vi "Motion Plot sub_VI.vi"(8 "Motion Parameters":T2={"Decel Time (s)"=0.0, "Accel Time (s)"=0.0, "Total Time (s)"=0.0, "Max Accel (mm/s^2)"=0.0, "Max Decel (mm/s^2)"=0.0, "Time step (s)"=0.01} {"Time step (s)" min=0.001}) -> (0 "Motion Points":T1, 1 "Accel Array":dbl[](graph), 2 "Velocity Array":dbl[](graph), 3 "Displacement Array":dbl[](graph), 4 "V max (mm/s)":dbl, 5 "Dist max (mm)":dbl)   [LabVIEW 2017]
panel:
  # "Use 0.01s"
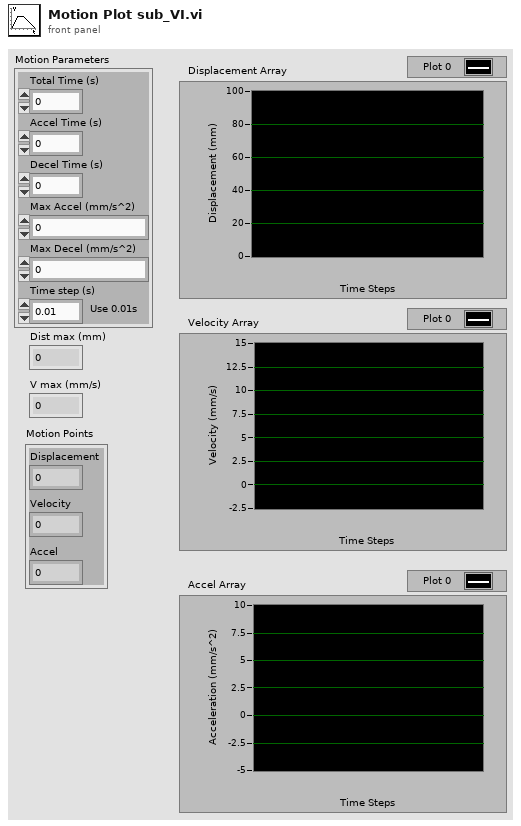
[diagram p1: front panel]
types:
  T1 = cluster{"Accel":dbl, "Velocity":dbl, "Displacement":dbl}
  T2 = cluster{"Decel Time (s)":dbl, "Accel Time (s)":dbl, "Total Time (s)":dbl, "Max Accel (mm/s^2)":dbl, "Max Decel (mm/s^2)":dbl, "Time step (s)":dbl}
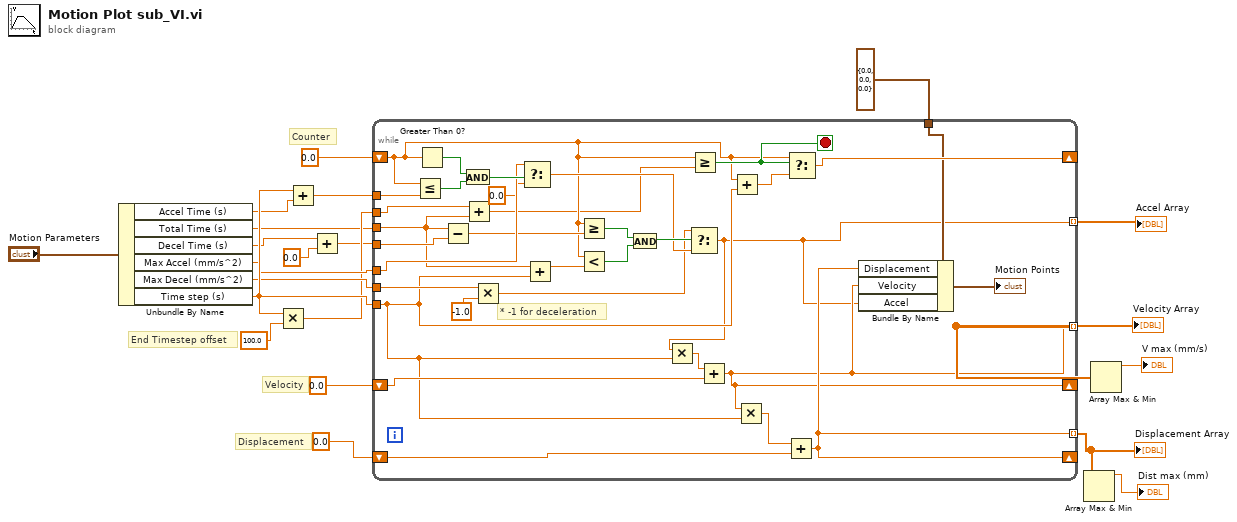
[diagram p0: block diagram]
diagram:
  # "End Timestep offset"
  # "Displacement"
  # "Velocity"
  # "Counter"
  n1 = Unbundle By Name("Motion Parameters") -> ("Accel Time (s)"=w4:dbl, "Total Time (s)"=w5:dbl, "Decel Time (s)"=w7:dbl, "Max Accel (mm/s^2)"=w17:dbl, "Max Decel (mm/s^2)"=w18:dbl, "Time step (s)"=w19:dbl)
  n2 = Multiply(x=w19, y=100.0) -> (x*y=w15:dbl)
  n3 = Add(x=w19, y=w4) -> (x+y=w11:dbl)
  n4 = Add(x=w7, y=0.0) -> (x+y=w12:dbl)
  n5 = while {
    shift-right: [w32] -> _
    shift-left: 0.0 -> [w31]
    tunnel: w11 -> [w54]
    tunnel: w17 -> [w50]
    tunnel: w5 -> [w42]
    tunnel: w12 -> [w47]
    tunnel: [w22] -> w6 mode=indexing
    tunnel: w18 -> [w34]
    shift-right: [w23] -> _
    shift-left: 0.0 -> [w39]
    shift-right: [w26] -> _
    shift-left: 0.0 -> [w37]
    tunnel: [w23] -> w20 mode=indexing
    tunnel: [w26] -> w3 mode=indexing
    tunnel: w19 -> [w29]
    tunnel: w15 -> [w27]
    tunnel: T1 {"Accel"=0.0, "Velocity"=0.0, "Displacement"=0.0} ("Motion Points 2") -> [w24]
    stop <- w40 stop-if-true
    # "* -1 for deceleration"
    n6 = Less Or Equal?(x=w31, y=w54) -> (x <= y?=w52:bool)
    n7 = Greater Than 0?(x=w31) -> (x > 0?=w53:bool)
    n8 = Subtract(x=w42, y=w47) -> (x-y=w48:dbl)
    n9 = And(x=w53, y=w52) -> (x .and. y?=w51:bool)
    n10 = Add(x=w27, y=w42) -> (x+y=w28:dbl)
    n11 = Multiply(x=w34, y=-1.0 ("x")) -> (x*y=w35:dbl)
    n12 = Select(t=w50, s=w51, f=0.0) -> (s? t:f=w43:dbl)
    n13 = Add(x=w42, y=w29) -> (x+y=w30:dbl)
    n14 = Greater Or Equal?(x=w31, y=w48) -> (x >= y?=w46:bool)
    n15 = Less?(x=w31, y=w30) -> (x < y?=w45:bool)
    n16 = And(x=w46, y=w45) -> (x .and. y?=w44:bool)
    n17 = Select(t=w35, s=w44, f=w43) -> (s? t:f=w22:dbl)
    n18 = Multiply(x=w22, y=w29) -> (x*y=w38:dbl)
    n19 = Greater Or Equal?(x=w31, y=w28) -> (x >= y?=w40:bool)
    n20 = Add(x=w38, y=w39) -> (x+y=w23:dbl)
    n21 = Add(x=w31, y=w29) -> (x+y=w41:dbl)
    n22 = Multiply(x=w23, y=w29) -> (x*y=w36:dbl)
    n23 = Add(x=w36, y=w37) -> (x+y=w26:dbl)
    n24 = Select(t=w31, s=w40, f=w41) -> (s? t:f=w32:dbl)
    n25 = Bundle By Name(cluster=w24, "Displacement"=w26, "Velocity"=w23, "Accel"=w22) -> (→"Motion Points":T1)
  }
  "Accel Array" <- w6
  "Velocity Array" <- w20
  "Displacement Array" <- w3
  n26 = Array Max & Min(array=w3) -> (max value=→"Dist max (mm)":dbl)  [unwired: 3 out]
  n27 = Array Max & Min(array=w20) -> (max value=→"V max (mm/s)":dbl)  [unwired: 3 out]
